vi "Transfer Group.Set Engine Offset.vi"(10 "engine offset":u64, 11 "Transfer Group in":refnum<class "Transfer Group.lvclass">) -> (3 "Transfer Group out":refnum<class "Transfer Group.lvclass">)   [LabVIEW 2017, in "DSF Core.lvlib" / "Transfer Group.lvclass"]
uses:
  Transfer Group.lvclass
  Transfer Group.lvclass/Transfer Group.ctl
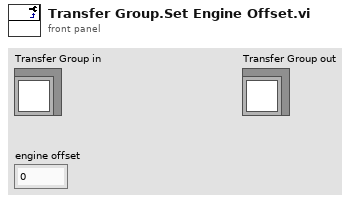
[diagram p1: front panel]
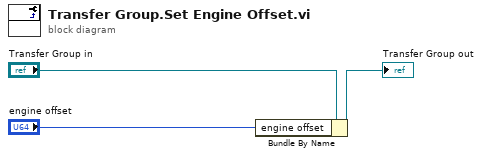
[diagram p0: block diagram]
diagram:
  n1 = Bundle By Name(cluster="Transfer Group in", "engine offset"="engine offset") -> (→"Transfer Group out":refnum<class "Transfer Group.lvclass">)
